vi "Yokogawa test.vi"() -> ()   [LabVIEW 2013]
panel:
  out "array":string[][](array[string])
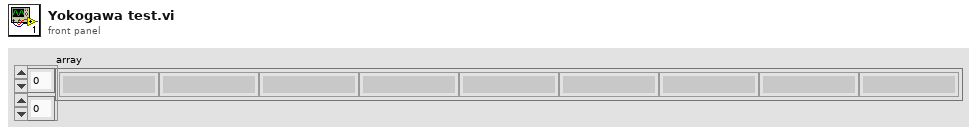
[diagram p1: front panel]
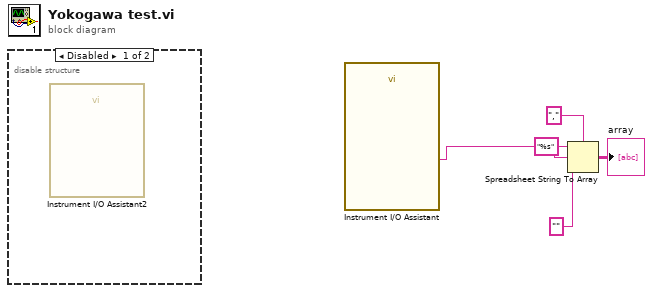
[diagram p0: block diagram]
diagram:
  n1 = disable-structure shown="Disabled" {
    frame Disabled {
      n2 = call "Instrument I/O Assistant2"() -> ()  [unwired: 25 in, 3 out]
    }
    frame Enabled {
    }
  }
  n3 = call "Instrument I/O Assistant"() -> ("token2"=w4:string)  [unwired: 25 in, 2 out]
  n4 = Spreadsheet String To Array(delimiter (Tab)=",", format string="%s", spreadsheet string=w4, array type (2D Dbl)="" ("delimiter (Tab)")) -> (array=→"array":string[][])
